vi "Hertz Amium.vi"(10 "Zeit [ms]":u32) -> (2 "Hertz":sgl)   [LabVIEW 2020, in "Amium PNS.lvlib" / "AK Kommunikation.lvlib"]
uses:
  AK Kommunikation.lvlib
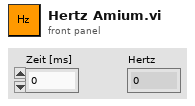
[diagram p1: front panel]
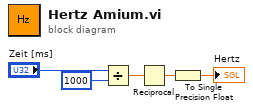
[diagram p0: block diagram]
diagram:
  n1 = Divide(x="Zeit [ms]", y=u32 1000) -> (x/y=w3:dbl)
  n2 = Reciprocal(x=w3) -> (1/x=w2:dbl)
  n3 = To Single Precision Float(number=w2) -> (single precision float=→"Hertz":sgl)
